vi "is_moving.vi"(7 "string":string, 8 "error in (no error)":errorcluster, 11 "client handle":T1) -> (0 "error out":errorcluster, 2 "moving":bool, 3 "client handle out":T1)   [LabVIEW 2022 SP3]
uses:
  <vilib>/httpClient/LabVIEWHTTPClient.lvlib
  <vilib>/httpClient/ClientHandle.ctl
panel:
  out "value":cluster{"status":i32}
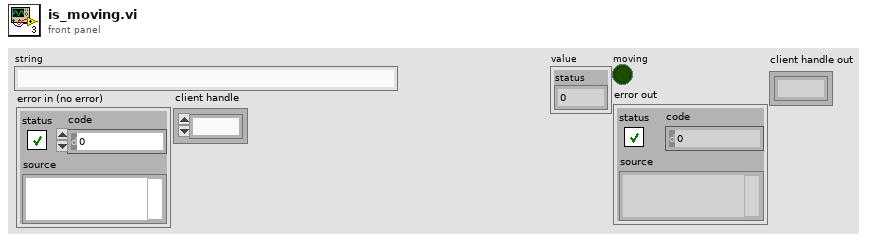
[diagram p1: front panel]
types:
  T1 = typedef "LabVIEWHTTPClient.lvlib/ClientHandle.ctl" = refnum<k1>
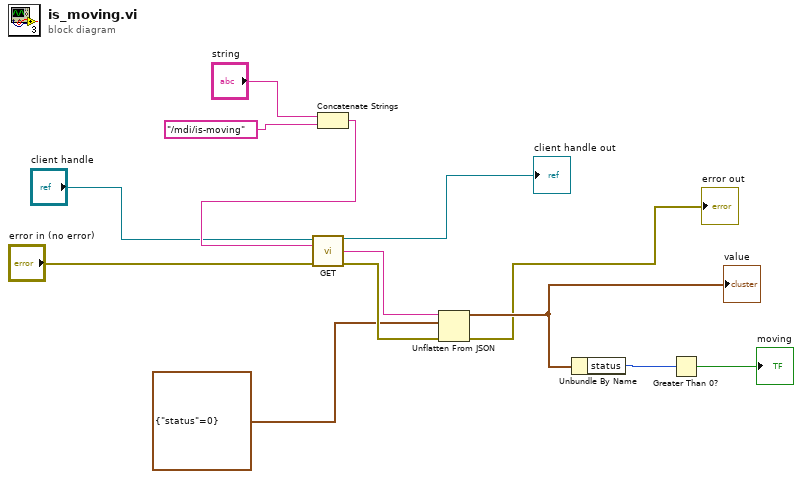
[diagram p0: block diagram]
diagram:
  n1 = Concatenate Strings("string", "/mdi/is-moving" ("string")) -> (w11:string)
  n2 = call <vilib>:"GET.vi"("client handle"="client handle", "url"=w11, "error in (no error)"="error in (no error)") -> ("client handle out"=→"client handle out":T1, "body"=w10:string, "error out"=w9:errorcluster)  [unwired: 9 in, 1 out]
  n3 = Unflatten From JSON(JSON string=w10, type and defaults=cluster{"status":i32} {"status"=0}, error in (no error)=w9) -> (value=w7:cluster{"status":i32}, error out=→"error out":errorcluster)  [unwired: 4 in]
  "value" <- w7
  n4 = Unbundle By Name(w7) -> ("status"=w6:i32)
  n5 = Greater Than 0?(x=w6) -> (x > 0?=→"moving":bool)
